vi "Do.vi"(8 "error in (no error)":errorcluster, 10 "Actor in":refnum<class "Actor.lvclass">, 11 "Configure Standard Waveform [STD] Msg":refnum<class "Configure Standard Waveform [STD] Msg.lvclass">) -> (0 "error out":errorcluster, 2 "Actor out":refnum<class "Actor.lvclass">)   [LabVIEW 2013, in "CS++Fgen.lvlib" / "Configure Standard Waveform [STD] Msg.lvclass"]
doc: "This VI delivers the message to the actor by calling the appropriate method(s) on the actor."
uses:
  Configure Standard Waveform [STD] Msg.lvclass
  <vilib>/ActorFramework/Actor/Actor.lvclass
  CS++Fgen/CS++Fgen.lvclass
  Configure Standard Waveform [STD] Msg.lvclass/Configure Standard Waveform [STD] Msg.ctl
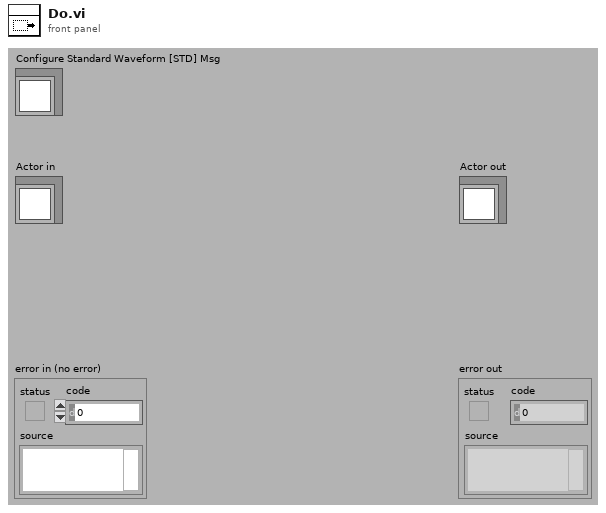
[diagram p1: front panel]
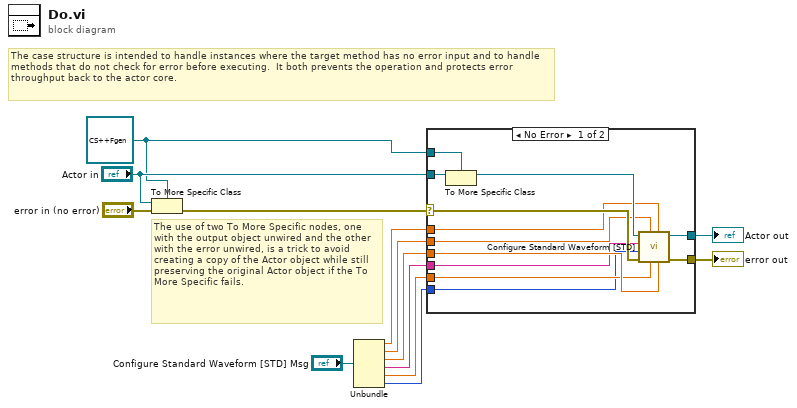
[diagram p0: block diagram]
diagram:
  w7 = refnum<class "CS++Fgen.lvclass"> refnum ("Actor in")
  # "The use of two To More Specific nodes, one with the output object unwired and the other with the error unwired, is a trick to avoid creating a copy of the Actor object while still preserving the original Actor object if the To More Specific fails."
  # "The case structure is intended to handle instances where the target method has no error input and to handle methods that do not check for error before executing.  It both prevents the operation and protects error throughput back to the actor core."
  n1 = To More Specific Class(target class=w7, reference="Actor in", error in="error in (no error)") -> (error out=w11:errorcluster)  [unwired: 1 out]
  n2 = Unbundle("Configure Standard Waveform [STD] Msg") -> (w6:dbl[unit], w5:dbl[unit], w4:dbl[unit], w3:string, w2:dbl[unit], w1:i32)
  n3 = case shown="No Error" w11 {
    selector: w11 -> [w23 w27]
    tunnel: [w25 w27] -> w10
    tunnel: [w24 w26] -> w9
    tunnel: "Actor in" -> [w22 w26]
    tunnel: w7 -> [w21 _]
    tunnel: w6 -> [w19 _]
    tunnel: w5 -> [w18 _]
    tunnel: w4 -> [w17 _]
    tunnel: w3 -> [w16 _]
    tunnel: w2 -> [w15 _]
    tunnel: w1 -> [w14 _]
    frame No Error {
      n4 = To More Specific Class(target class=w21, reference=w22) -> (specific class reference=w20:refnum<class "CS++Fgen.lvclass">)  [unwired: 1 in, 1 out]
      n5 = call "Configure Standard Waveform [STD].vi"("dc offset (0.00 V)"=w17, "start phase (0.00 Degrees)"=w19, "amplitude (1.00 V)"=w15, "frequency (1000.0 Hz)"=w18, "error in (no error)"=w23, "waveform (Sine)"=w14, "channel name (\"CHANNEL1\")"=w16, "CS++Fgen in"=w20) -> ("error out"=w25:errorcluster, "CS++Fgen out"=w24:refnum<class "CS++Fgen.lvclass">)  [unwired: 2 in]
    }
    frame Error {
      # "If type check fails, pass the original object out again."
    }
  }
  "error out" <- w10
  "Actor out" <- w9
